vi "test anything ti bdbl.vi"() -> ()   [LabVIEW 2019]
panel:
  out "DBL_ARR":dbl[](array[numeric])
  out "NAME_ARR":string[](array[string])
  in  "x":T1
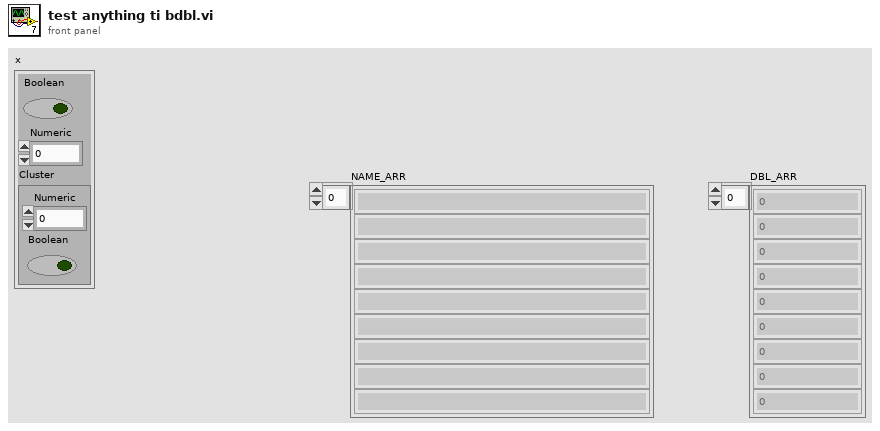
[diagram p1: front panel]
types:
  T1 = cluster{"Boolean":bool, "Numeric":dbl, "Cluster":cluster{"Numeric":dbl, "Boolean":bool}}
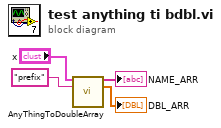
[diagram p0: block diagram]
diagram:
  n1 = call "AnyThingToDoubleArray.vi"("Claster"="x", "Prefix"="prefix") -> ("NAME_ARR"=→"NAME_ARR":string[], "DBL_ARR"=→"DBL_ARR":dbl[])  [unwired: 11 in, 1 out]
